vi "Determine if Executable.vi"(1 "Path":path) -> (0 "EXE?":bool)   [LabVIEW 2023]
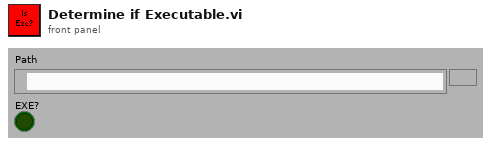
[diagram p1: front panel]
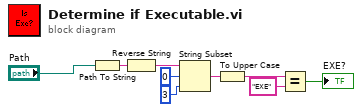
[diagram p0: block diagram]
diagram:
  n1 = Path To String(path="Path") -> (string=w9:string)
  n2 = Reverse String(1:w9) -> (0:w8:string)
  n3 = String Subset(string=w8, offset (0)=0, length (rest)=3 ("length (rest)")) -> (substring=w5:string)
  n4 = To Upper Case(1:w5) -> (0:w4:string)
  n5 = Equal?(x=w4, y="EXE") -> (x = y?=→"EXE?":bool)
